vi "PWM signal.vi"(8 "Signo":bool, 9 "Amplitud":dbl(knob) scale=0.0..6.0, 10 "Ciclo de trabajo":dbl(knob) scale=0.0..100.0, 11 "Frecuencia":dbl(knob) scale=0.0..30.0) -> (2 "Waveform Chart":dbl(graph))   [LabVIEW 2018]
doc: "Crea una señal PWM ajustable mediante sus entradas ciclo de trabajo, frecuencia y amplitud"
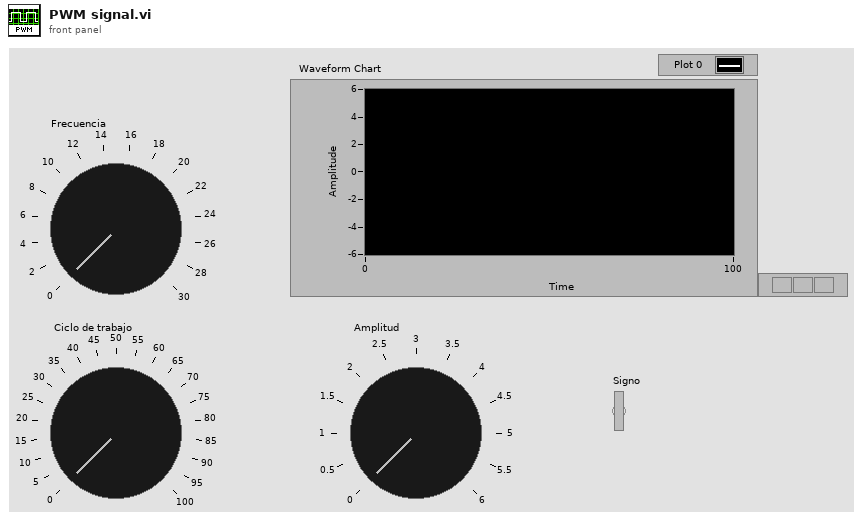
[diagram p1: front panel]
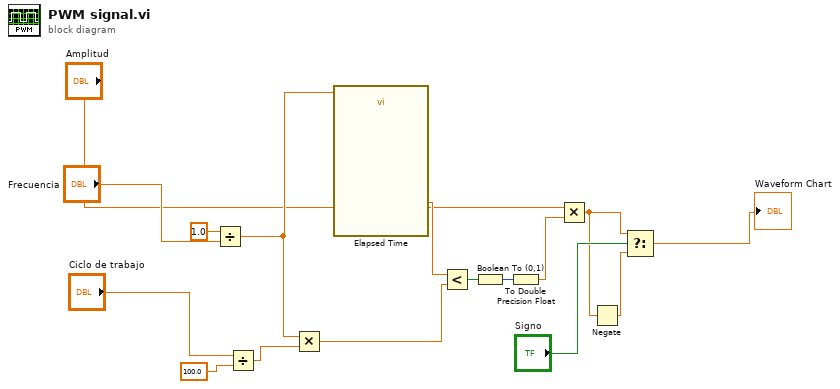
[diagram p0: block diagram]
diagram:
  n1 = Divide(x=1.0, y="Frecuencia") -> (x/y=w7:dbl)
  n2 = Divide(x="Ciclo de trabajo", y=100.0) -> (x/y=w8:dbl)
  n3 = Multiply(x=w7, y=w8) -> (x*y=w6:dbl)
  n4 = call "Elapsed Time"("Time Target (s)"=w7) -> ("Elapsed Time (s)"=w14:dbl)  [unwired: 11 in, 7 out]
  n5 = Less?(x=w14, y=w6) -> (x < y?=w13:bool)
  n6 = Boolean To (0,1)(Boolean=w13) -> (0, 1=w12:i16)
  n7 = To Double Precision Float(number=w12) -> (double precision float=w11:dbl)
  n8 = Multiply(x="Amplitud", y=w11) -> (x*y=w2:dbl)
  n9 = Negate(x=w2) -> (-x=w3:dbl)
  n10 = Select(t=w2, s="Signo", f=w3) -> (s? t:f=→"Waveform Chart":dbl)
